vi "Request Sink by Name.vi"(8 "error in (no error)":errorcluster, 10 "Sink Name":string, 11 "Sink Look Up Table in":refnum<class "Sink Look Up Table.lvclass">) -> (0 "error out":errorcluster, 1 "Found?":bool, 2 "Log Sink":refnum<data-value>, 3 "Sink Look Up Table out":refnum<class "Sink Look Up Table.lvclass">)   [LabVIEW 2016, in "Stream Log.lvlib" / "Sink Look Up Table.lvclass"]
doc: "--\nCopyright © 2017 Composed SystemsI All rights reserved.\n\nAuthor: Jon McBee <jon.mcbee@composed.io>\n\nThis library is provided \"AS IS\" ,WITHOUT WARRANTIES OR\nCONDITIONS OF ANY KIND, either express or implied.\n\nComposed Systems -- composed.io\n\nStream 0.0.1.1\nJon McBee - Composed Systems\nCopyright (c) 2017, Composed Systems"
uses:
  <userlib>/Composed Systems/Stream/Log/Sink Look Up Table/Sink Look Up Table.lvclass
  C:/Program Files (x86)/National Instruments/LabVIEW 2016/user.lib/Composed Systems/Stream/Look Up Table/Look Up Table/Look Up Table.lvclass
  <userlib>/Composed Systems/Stream/Log/Log Sink/Log Sink.lvclass
  <userlib>/Composed Systems/Stream/Look Up Table/Look Up Table/Look Up Table.lvclass
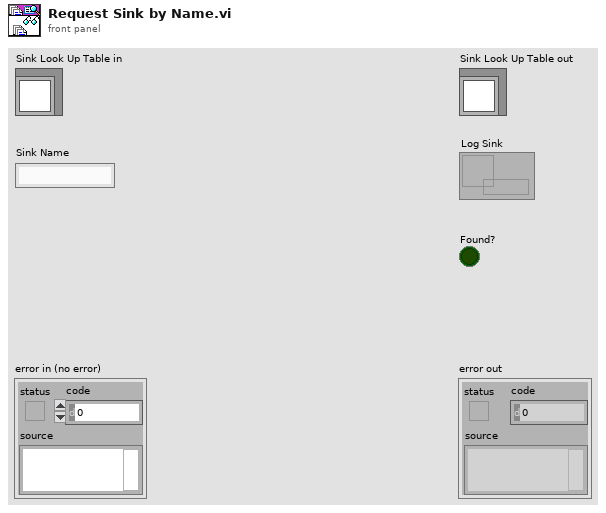
[diagram p1: front panel]
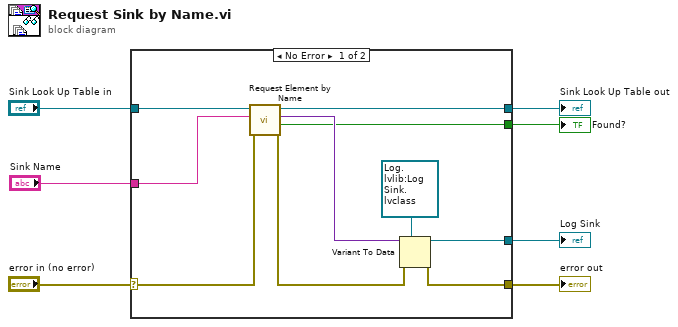
[diagram p0: block diagram]
diagram:
  n1 = case shown="No Error" "error in (no error)" {
    selector: "error in (no error)" -> [w14 w19]
    tunnel: [w11 w19] -> w6
    tunnel: [w16 w18] -> w4
    tunnel: "Sink Look Up Table in" -> [w17 w18]
    tunnel: "Sink Name" -> [w15 _]
    tunnel: [w9 _] -> w2
    tunnel: [w8 _] -> w1
    frame No Error {
      n2 = call <userlib>:"Request Element by Name.vi"("error in (no error)"=w14, "Name"=w15, "Look Up Table in"=w17) -> ("error out"=w12:errorcluster, "Found?"=w9:bool, "Element"=w13:variant, "Look Up Table out"=w16:refnum<class "Sink Look Up Table.lvclass">)  [unwired: 5 in]
      n3 = Variant To Data(error in=w12, type=refnum<data-value> refnum ("Log Sink"), Variant=w13) -> (data=w8:refnum<data-value>, error out=w11:errorcluster)
    }
    frame Error {
    }
  }
  "error out" <- w6
  "Sink Look Up Table out" <- w4
  "Found?" <- w2
  "Log Sink" <- w1
